vi "NI VeriStand - Stop Data Logging.vi"(8 "error in (no error)":errorcluster, 10 "Data Log Configuration Name":string, 11 "WorkspaceManager in":T1) -> (0 "error out":errorcluster, 3 "WorkspaceManager out":T1)   [LabVIEW 2020, in "NI_VS Workspace ExecutionAPI.lvlib"]
doc: "Stops logging data for the specified <B>Data Log Configuration Name</B>."
uses:
  <vilib>/NI VeriStand/Execution/Workspace/NI_VS Workspace ExecutionAPI.lvlib
  <vilib>/NI VeriStand/Execution/Workspace/WorkspaceAPI.ctl
  NationalInstruments.VeriStand.ClientAPI
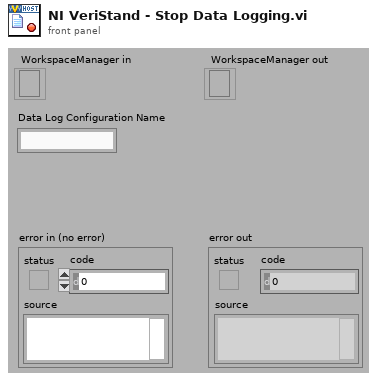
[diagram p1: front panel]
types:
  T1 = typedef "NI_VS Workspace ExecutionAPI.lvlib/WorkspaceAPI.ctl" = refnum<k24>
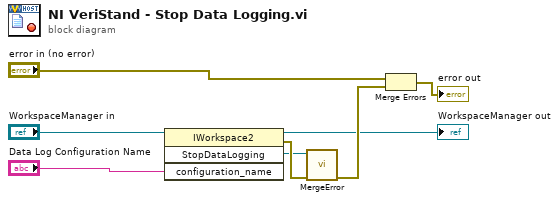
[diagram p0: block diagram]
diagram:
  n1 = invoke class="IWorkspace2" method="StopDataLogging"(reference="WorkspaceManager in", "configuration_name"="Data Log Configuration Name") -> (reference out=→"WorkspaceManager out":T1, error out=w8:errorcluster, "StopDataLogging"=w6:refnum<k24>)  [unwired: 2 in, 1 out]
  n2 = call <vilib>:"MergeError.vi"("error in (no error)"=w8, "Error"=w6) -> ("error out"=w7:errorcluster)  [unwired: 9 out]
  n3 = Merge Errors("error in (no error)", w7) -> (→"error out":errorcluster)
